vi "Temperature Write Single.vi"(8 "error in":errorcluster, 9 "Channel Index":i32=1, 10 "Temperature AV":dbl, 11 "Climate Chamber in":refnum<class "Climate Chamber.lvclass">) -> (0 "error out":errorcluster, 3 "Climate Chamber out":refnum<class "Climate Chamber.lvclass">)   [LabVIEW 2023, in "Climate Chamber.lvclass"]
uses:
  Climate Chamber.lvclass
  Low Level Capabilities/Temperature/Temperature Actual Value/Temperature Actual Value.lvclass
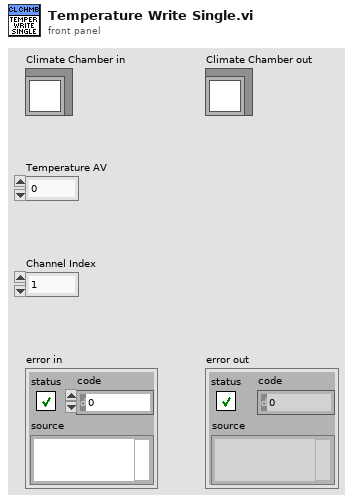
[diagram p1: front panel]
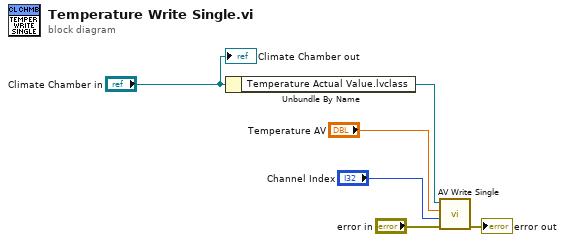
[diagram p0: block diagram]
diagram:
  n1 = Unbundle By Name("Climate Chamber in") -> ("Temperature Actual Value.lvclass"=w5:refnum<class "Temperature Actual Value.lvclass">)
  n2 = call-dynamic "AV Write Single.vi"("error in"="error in", "Channel Index"="Channel Index", "Temperature AV"="Temperature AV", "Temperature Actual Value in"=w5) -> ("error out"=→"error out":errorcluster)  [unwired: 6 in, 1 out]
  "Climate Chamber out" <- "Climate Chamber in"
